vi "Init.vi"(9 "Max Time":u8=24, 10 "Blueprint String":string, 11 "Blueprint in":refnum<class "Blueprint.lvclass">) -> (3 "Blueprint out":refnum<class "Blueprint.lvclass">)   [LabVIEW 2023, in "d19.lvlib" / "Blueprint.lvclass"]
uses:
  Blueprint/Blueprint.lvclass
  Blueprint/Blueprint.lvclass/Blueprint.ctl
  Mine/Mine.lvclass
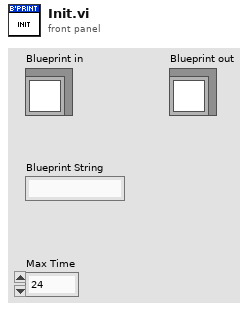
[diagram p1: front panel]
types:
  T1 = cluster{"Ore Robot Ore Cost":u8, "Clay Robot Ore Cost":u8, "Obsidian Robot Ore Cost":u8, "Geode Robot Ore Cost":u8, "Obsidian Robot Clay Cost":u8, "Geode Robot Obsidian Cost":u8}
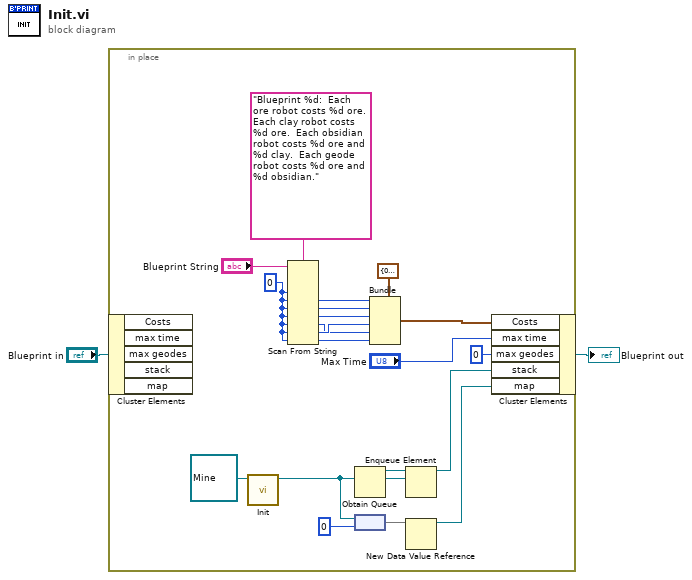
[diagram p0: block diagram]
diagram:
  n1 = in-place {
    w20 = u8 0 ("default value 1")
    n2 = in-place-cluster #1("Blueprint in") -> ()  [unwired: 5 out]
    n3 = call "Init.vi"("Mine in"=refnum<class "Mine.lvclass"> refnum ("d19.lvlib:Robots.lvclass")) -> ("Mine out"=w4:refnum<class "Mine.lvclass">)  [unwired: 10 in]
    n4 = Scan From String(format string="Blueprint %d:  Each ore robot costs %d ore.  Each clay robot costs %d ore.  Each obsidian robot costs %d ore and %d clay.  Each geode robot costs %d ore and %d obsidian.", input string="Blueprint String", default 1=w20, default 2=w20, default 3=w20, default 4=w20, default 5=w20, default 6=w20, default 7=w20) -> (output 2=w18:u8, output 3=w17:u8, output 4=w16:u8, output 5=w14:u8, output 6=w15:u8, output 7=w13:u8)  [unwired: 3 in, 3 out]
    n5 = Obtain Queue(element data type=w4) -> (queue out=w8:refnum<queue>)  [unwired: 4 in, 2 out]
    n6 = node(w4, u8 0 ("value")) -> (w6:map{refnum<class "Mine.lvclass">, u8})
    n7 = Bundle(cluster=T1 {"Ore Robot Ore Cost"=0, "Clay Robot Ore Cost"=0, "Obsidian Robot Ore Cost"=0, "Geode Robot Ore Cost"=0, "Obsidian Robot Clay Cost"=0, "Geode Robot Obsidian Cost"=0} ("Costs"), "Ore Robot Ore Cost"=w18, "Clay Robot Ore Cost"=w17, "Obsidian Robot Ore Cost"=w16, "Geode Robot Ore Cost"=w15, "Obsidian Robot Clay Cost"=w14, "Geode Robot Obsidian Cost"=w13) -> (w12:T1)
    n8 = Enqueue Element(queue=w8, element=w4) -> (queue out=w5:refnum<queue>)  [unwired: 2 in, 2 out]
    n9 = New Data Value Reference(data value=w6) -> (data value reference=w3:refnum<data-value>)  [unwired: 1 in, 1 out]
    n10 = in-place-cluster #1("Costs"=w12, "max time"="Max Time", "max geodes"=u8 0, "stack"=w5, "map"=w3) -> (→"Blueprint out":refnum<class "Blueprint.lvclass">)
  }
